vi "Symmetrize (multiple).vi"(8 "error in (no error)":errorcluster, 11 "XY-data":cluster{"X-array":dbl[], "Y-array":dbl[]}[](array[cluster]) {"Y-array" format="%.2p"; "X-array" format="%.2p"}) -> (0 "error out":errorcluster, 1 "Antisymmetric":cluster{"X-array":dbl[], dbl[]}[](array[cluster]), 2 "Symmetric":cluster{"X-array":dbl[], dbl[]}[](array[cluster]), 3 "XY-data out":cluster{"X-array":dbl[], "Y-array":dbl[]}[](array[cluster]) {"Y-array" format="%.2p"; "X-array" format="%.2p"})   [LabVIEW 2019, in "xy_utilities.lvlib"]
doc: "Compute the Symmetric and Antisymmetric functions of <b>XY-data</b>\n\n<b>Symmetric</b>: f+ = (f(x) + f(-x))/2\n<b>Antisymmetric</b>: f- = (f(x) - f(-x))/2"
uses:
  xy_utilities.lvlib
  Sort.vi
  Sort (single).vi
  <userlib>/_OpenG.lib/array/array.llb/Sort Array__ogtk.vi
  <userlib>/_OpenG.lib/array/array.llb/Sort 1D Array (DBL)__ogtk.vi
  <userlib>/_OpenG.lib/array/array.llb/Reorder Array2__ogtk.vi
  <userlib>/_OpenG.lib/array/array.llb/Reorder 1D Array2 (DBL)__ogtk.vi
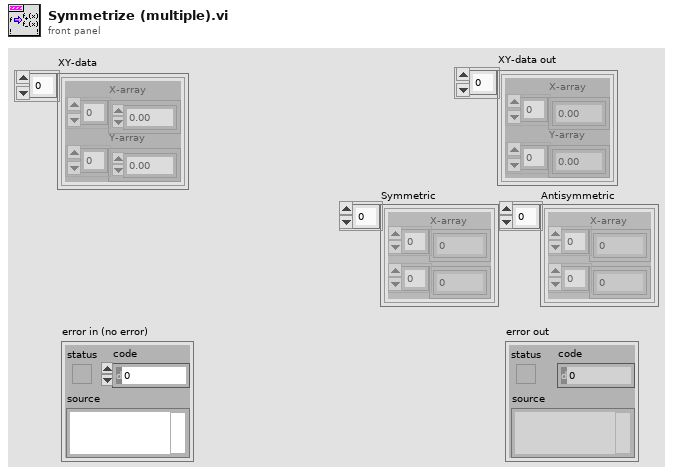
[diagram p1: front panel]
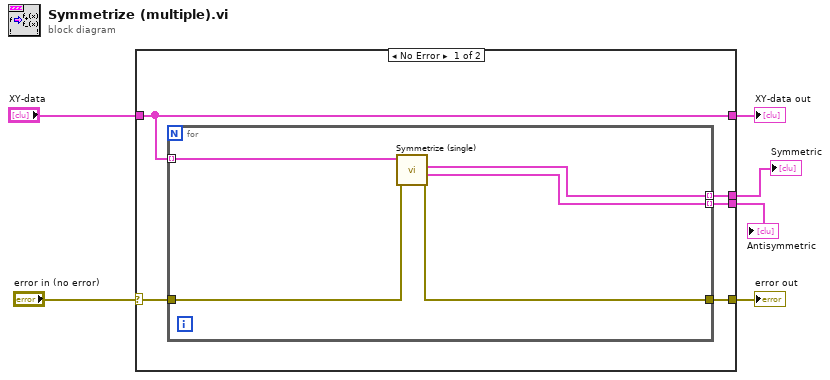
[diagram p0: block diagram]
diagram:
  n1 = case shown="No Error" "error in (no error)" {
    selector: "error in (no error)" -> [w9 w18]
    tunnel: [w8 w18] -> w5
    tunnel: "XY-data" -> [w7 w17]
    tunnel: [w7 w17] -> w3
    tunnel: [w11 _] -> w2
    tunnel: [w10 _] -> w1
    frame No Error {
      n2 = for {
        tunnel: w7 -> [w16] mode=indexing
        tunnel: [w15] -> w11 mode=indexing
        tunnel: [w14] -> w10 mode=indexing
        tunnel: w9 -> [w12]
        tunnel: [w13] -> w8
        n3 = call "Symmetrize (single).vi"("error in (no error)"=w12, "XY-data"=w16) -> ("error out"=w13:errorcluster, "Antisymmetric"=w14:cluster{"X-array":dbl[], dbl[]}, "Symmetric"=w15:cluster{"X-array":dbl[], dbl[]})  [unwired: 6 in, 1 out]
      }
    }
    frame Error {
    }
  }
  "error out" <- w5
  "XY-data out" <- w3
  "Symmetric" <- w2
  "Antisymmetric" <- w1
